vi "U64toU32.vi"(6 "ready for output":bool, 9 "input valid":bool, 11 "U64 in":u64) -> (1 "output valid":bool, 3 "U32 out":u32, 4 "ready for input":bool)   [LabVIEW 2016]
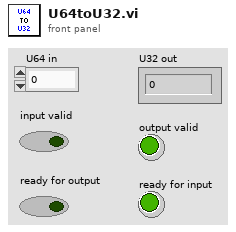
[diagram p1: front panel]
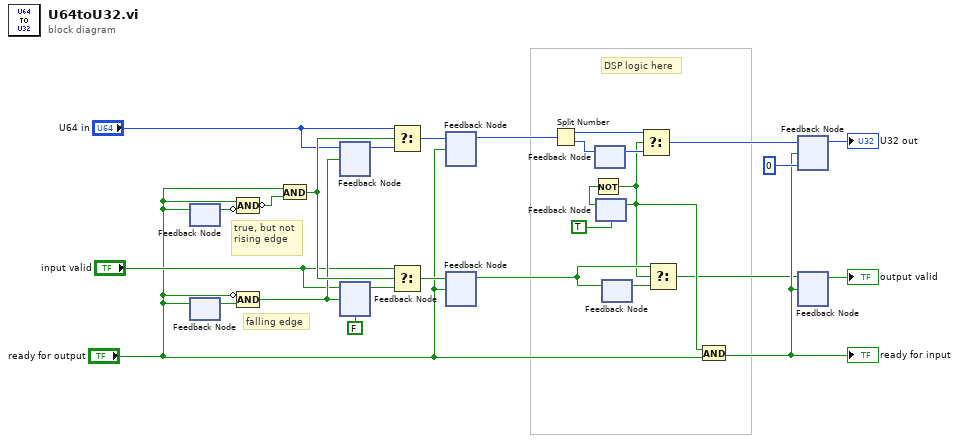
[diagram p0: block diagram]
diagram:
  # "DSP logic here"
  # "falling edge"
  # "true, but not rising edge"
  n1 = feedback #1() -> (w15:bool)  [unwired: 1 in]
  n2 = feedback-in #1("ready for output") -> ()
  n3 = feedback #2() -> (w16:bool)  [unwired: 1 in]
  n4 = feedback-in #2("ready for output") -> ()
  n5 = Compound Arithmetic op=AND("ready for output", invert w15) -> (invert w14:bool)
  n6 = Compound Arithmetic op=AND(invert "ready for output", w16) -> (w19:bool)
  n7 = And(x="ready for output", y=w14) -> (x .and. y?=w20:bool)
  n8 = feedback #3() -> (w13:u64)  [unwired: 1 in]
  n9 = feedback-in #3("U64 in", w19) -> ()
  n10 = feedback #4(FALSE) -> (w17:bool)
  n11 = feedback-in #4("input valid", w19) -> ()
  n12 = Select(t="U64 in", s=w20, f=w13) -> (s? t:f=w22:u64)
  n13 = Select(t="input valid", s=w20, f=w17) -> (s? t:f=w23:bool)
  n14 = feedback #5() -> (w25:u64)  [unwired: 1 in]
  n15 = feedback-in #5(w22, "ready for output") -> ()
  n16 = feedback #6() -> (w3:bool)  [unwired: 1 in]
  n17 = feedback-in #6(w23, "ready for output") -> ()
  n18 = Split Number(x=w25) -> (hi(x)=w10:u32, lo(x)=w8:u32)
  n19 = feedback #7() -> (w9:u32)  [unwired: 1 in]
  n20 = feedback-in #7(w8) -> ()
  n21 = feedback #8(TRUE) -> (w7:bool)
  n22 = Not(x=w7) -> (.not. x?=w2:bool)
  n23 = feedback-in #8(w2) -> ()
  n24 = feedback #9() -> (w4:bool)  [unwired: 1 in]
  n25 = feedback-in #9(w3) -> ()
  n26 = Select(t=w10, s=w2, f=w9) -> (s? t:f=w27:u32)
  n27 = Select(t=w3, s=w2, f=w4) -> (s? t:f=w1:bool)
  n28 = And(x=w2, y="ready for output") -> (x .and. y?=w5:bool)
  "ready for input" <- w5
  n29 = feedback #10(u32 0 ("(hi.lo)")) -> (→"U32 out":u32)
  n30 = feedback-in #10(w27, w5) -> ()
  n31 = feedback #11() -> (→"output valid":bool)  [unwired: 1 in]
  n32 = feedback-in #11(w1, w5) -> ()
